vi "pid demo integrator.vi"(1 "delta t":dbl format="%.2f", 3 "input":dbl format="%.2f", 4 "gain":dbl=1.0 format="%.2f") -> (5 "output":dbl format="%.2f")   [LabVIEW 2016]
doc: "This subVI performs integration using the Trapezoidal Rule."
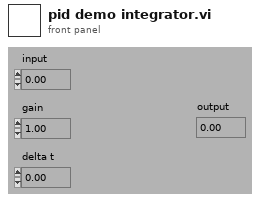
[diagram p1: front panel]
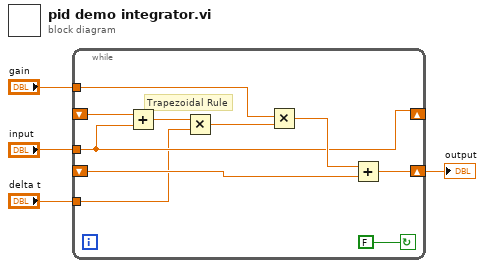
[diagram p0: block diagram]
diagram:
  n1 = while {
    shift-left: _ -> [w12]
    shift-right: [w11] -> w1
    tunnel: "gain" -> [w14]
    tunnel: "input" -> [w9]
    tunnel: "delta t" -> [w7]
    shift-left: _ -> [w10]
    shift-right: [w9] -> _
    stop <- FALSE continue-if-true
    # "Trapezoidal Rule"
    n2 = Add(x=w10, y=w9) -> (x+y=w8:dbl)
    n3 = Multiply(x=w8, y=w7) -> (x*y=w6:dbl)
    n4 = Multiply(x=w14, y=w6) -> (x*y=w13:dbl)
    n5 = Add(x=w13, y=w12) -> (x+y=w11:dbl)
  }
  "output" <- w1
